vi "Enqueue.vi"(8 "error in (no error)":errorcluster, 9 "Data":variant, 10 "Command":string, 11 "Queue In":T1) -> (0 "error out":errorcluster, 3 "Queue Out":T1)   [LabVIEW 2023, in "Internal Communication.lvlib"]
uses:
  Internal Communication.lvlib
  Controls/Queue.ctl
  Controls/Base Message.ctl
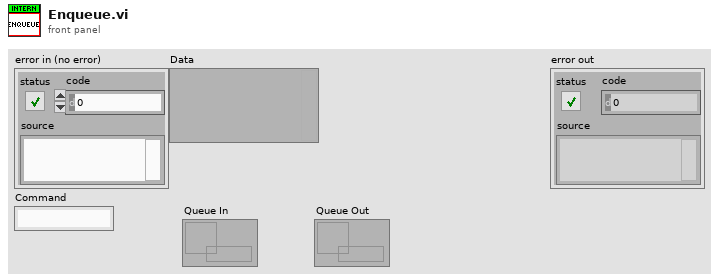
[diagram p1: front panel]
types:
  T1 = typedef "Queue.ctl" = refnum<queue>
  T2 = typedef "Internal Communication.lvlib/Base Message.ctl" = cluster{"Command":string, "Data":variant}
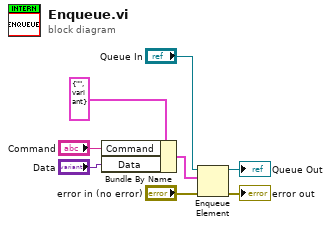
[diagram p0: block diagram]
diagram:
  n1 = Bundle By Name(cluster=T2 {"Command"="", "Data"=variant} ("Message"), "Command"="Command", "Data"="Data") -> (w1:T2)
  n2 = Enqueue Element(queue="Queue In", element=w1, error in (no error)="error in (no error)") -> (queue out=→"Queue Out":T1, error out=→"error out":errorcluster)  [unwired: 1 in, 1 out]
